vi "myRIO_BRig_RT__Case_Exp_State_initBlock2.vi"(7 "input_spout":enum16{"Left", "Right"}(ring), 9 "input_dataBlock":u16[][](array[numeric]), 11 "input_dataCurrent":u16[](array[numeric])) -> (0 "idxDataBlock":i32, 1 "output_dataBlock":u16[][](array[numeric]))   [LabVIEW 2014]
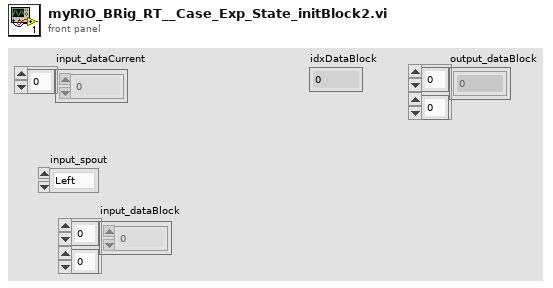
[diagram p1: front panel]
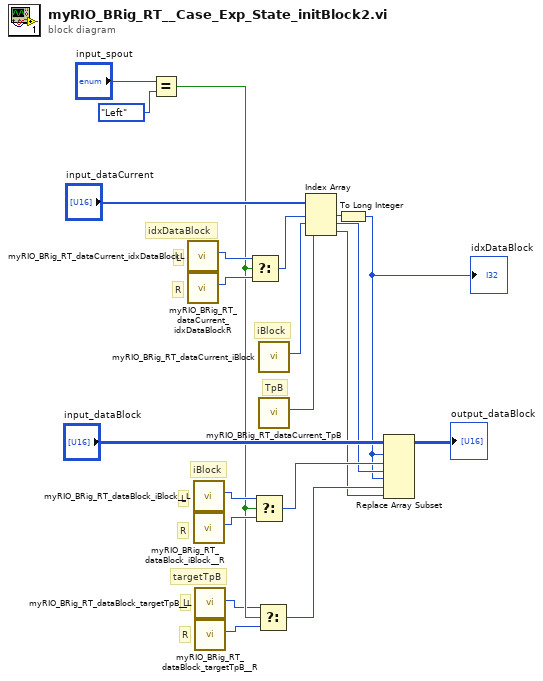
[diagram p0: block diagram]
diagram:
  # "TpB"
  # "iBlock"
  # "R"
  # "L"
  # "targetTpB"
  # "R"
  # "L"
  # "idxDataBlock"
  # "R"
  # "L"
  # "iBlock"
  n1 = Equal?(x="input_spout", y=enum16{"Left", "Right"}."Left") -> (x = y?=w13:bool)
  n2 = call "myRIO_BRig_RT_dataCurrent_idxDataBlockL.vi"() -> ("output_idxDataBlock__L"=w18:i32)  [unwired: 11 in]
  n3 = call "myRIO_BRig_RT_dataCurrent_idxDataBlockR.vi"() -> ("output_idxDataBlock__R"=w17:i32)  [unwired: 11 in]
  n4 = call "myRIO_BRig_RT_dataBlock_iBlock__L.vi"() -> ("output_iBlock__L"=w15:i32)  [unwired: 11 in]
  n5 = call "myRIO_BRig_RT_dataBlock_iBlock__R.vi"() -> ("output_iBlock__R"=w14:i32)  [unwired: 11 in]
  n6 = call "myRIO_BRig_RT_dataBlock_targetTpB__L.vi"() -> ("output_targetTpB__L"=w12:i32)  [unwired: 11 in]
  n7 = call "myRIO_BRig_RT_dataBlock_targetTpB__R.vi"() -> ("output_targetTpB__R"=w11:i32)  [unwired: 11 in]
  n8 = Select(t=w18, s=w13, f=w17) -> (s? t:f=w2:i32)
  n9 = Select(t=w15, s=w13, f=w14) -> (s? t:f=w9:i32)
  n10 = Select(t=w12, s=w13, f=w11) -> (s? t:f=w8:i32)
  n11 = call "myRIO_BRig_RT_dataCurrent_iBlock.vi"() -> ("output_iBlock"=w7:i32)  [unwired: 11 in]
  n12 = call "myRIO_BRig_RT_dataCurrent_TpB.vi"() -> ("output_TpB"=w6:i32)  [unwired: 11 in]
  n13 = Index Array(array="input_dataCurrent", index #1=w2, index #2=w7, index #3=w6) -> (element #1=w10:u16, element #2=w5:u16, element #3=w4:u16)
  n14 = To Long Integer(number=w10) -> (32bit integer=w1:i32)
  "idxDataBlock" <- w1
  n15 = Replace Array Subset(array="input_dataBlock", new element #1=w5, index (row) #1=w1, index (col) #1=w9, new element #2=w4, index (row) #2=w1, index (col) #2=w8) -> (→"output_dataBlock":u16[][])
